vi "Initialize.vi"(7 "Serial Configuration":T1={"Baud Rate"=9600, "Parity"=0, "Data Bits"=8, "Stop Bits"=10, "Flow Control"=0} {"Flow Control" items=["None", "XON/XOFF", "RTS/CTS", "XON/XOFF & RTS/CTS", "DTR/DSR", "XON/XOFF & DTR/DSR"]; "Stop Bits" items=["1.0"=10, "1.5"=15, "2.0"=20]; "Data Bits" items=["7"=7, "8"=8]; "Parity" items=["None", "Odd", "Even", "Mark", "Space"]; "Baud Rate" items=["300"=300, "600"=600, "1200"=1200, "2400"=2400, "4800"=4800, "9600"=9600, "19200"=19200]}, 8 "error in (no error)":errorcluster, 9 "Reset (True)":bool=TRUE, 10 "ID Query (True)":bool=TRUE, 11 "VISA resource name":refnum<visa-resource-name>) -> (0 "error out":errorcluster, 3 "VISA resource name out":refnum<visa-resource-name>)   [LabVIEW 2020, in "Keithley 24XX.lvlib"]
doc: "Establishes communication with the instrument and optionally performs an instrument identification query and/or an instrument reset. It also places the instrument in a default state needed for other instrument driver operations. Therefore, call this VI before calling other instrument driver VIs for this instrument. Generally, you need to call the Initialize VI only once at the beginning of an application."
uses:
  Keithley 24XX.lvlib
panel:
  # "(c) 2006 - 2015 National Instruments.  ALL RIGHTS RESERVED."
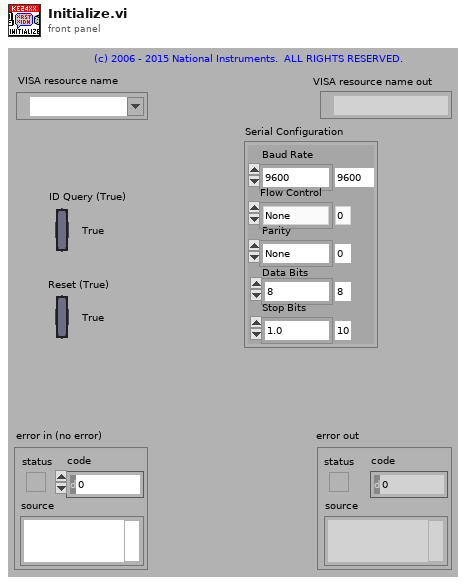
[diagram p1: front panel]
types:
  T1 = cluster{"Baud Rate":u32, "Parity":u16, "Data Bits":u16, "Stop Bits":u16, "Flow Control":u16}
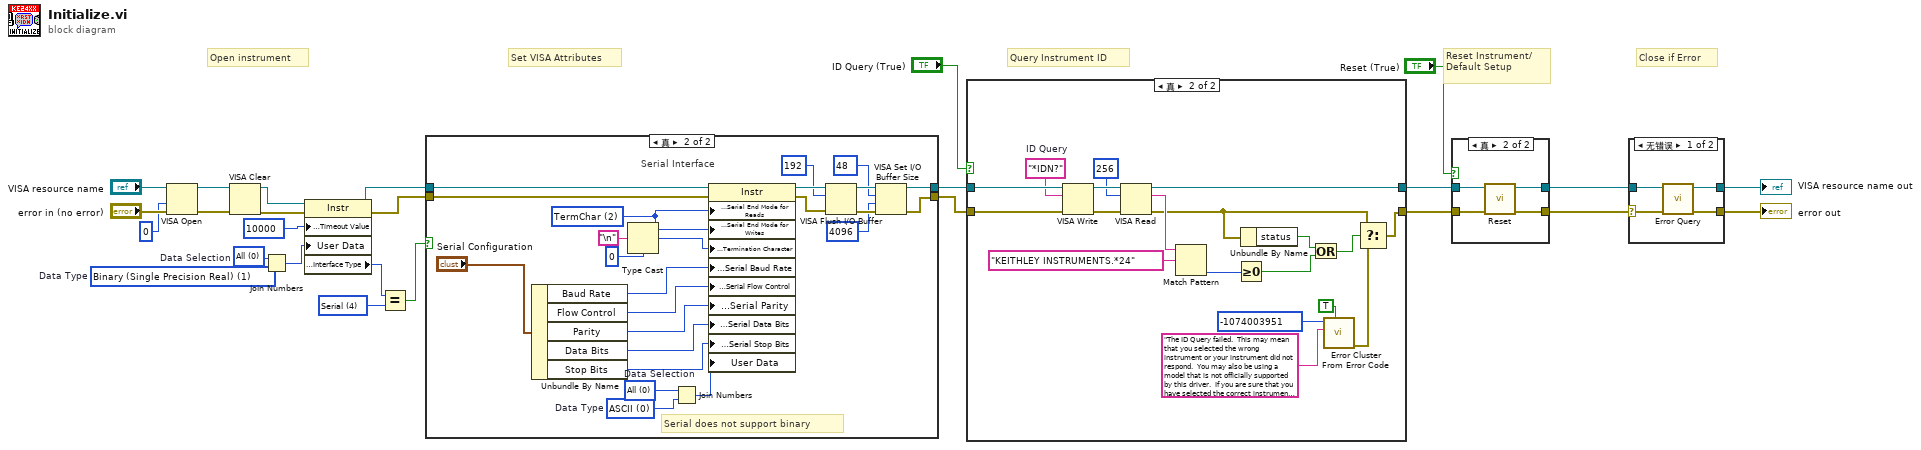
[diagram p0: block diagram]
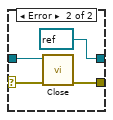
[diagram p3: hidden frame]
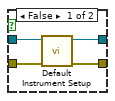
[diagram p4: hidden frame]
diagram:
  w2 = u16 1 items=["ASCII", "Binary (Single Precision Real)"]  # Data Type
  w3 = u16 0 items=["All", "Volt and Amp", "Volt", "Amp"]  # Data Selection
  w14 = u16 4 items=["GPIB"=1, "VXI"=2, "GPIB-VXI"=3, "Serial"=4, "PXI"=5, "TCPIP"=6, "USB"=7] ("Interface Information:Interface Type")
  # "Set VISA Attributes"
  # "Close if Error"
  # "Query Instrument ID"
  # "Reset Instrument/\nDefault Setup"
  # "Open instrument"
  n1 = VISA Open(access mode=u32 0, error in (no error)="error in (no error)", VISA resource name="VISA resource name") -> (VISA resource name=w12:refnum<visa-resource-name>, error out=w11:errorcluster)  [unwired: 2 in]
  n2 = VISA Clear(VISA resource name=w12, error in (no error)=w11) -> (VISA resource name out=w10:refnum<visa-resource-name>, error out=w9:errorcluster)
  n3 = Join Numbers(hi=w3, lo=w2) -> ((hi.lo)=w1:u32)
  n4 = property class="Instr"(reference=w10, error in=w9, "General Settings:Timeout Value"=u32 10000, "User Data"=w1) -> (reference out=w17:refnum<visa-resource-name>, error out=w16:errorcluster, "Interface Information:Interface Type"=w4:u16)
  n5 = Equal?(x=w4, y=w14) -> (x = y?=w15:bool)
  n6 = case shown="真" w15 {
    tunnel: [w27 w49] -> w19
    tunnel: [w28 w46] -> w18
    tunnel: w17 -> [w27 w51]
    tunnel: w16 -> [w28 w52]
    frame False {
      # "GPIB"
    }
    frame True {
      w31 = u16 0 items=["ASCII", "Binary (Single Precision Real)"]  # Data Type
      w29 = u16 0 items=["All", "Volt and Amp", "Volt", "Amp"]  # Data Selection
      w39 = u16 2 items=["None", "LastBit", "TermChar"] ("Serial Settings:Serial End Mode for Reads")
      # "Serial does not support binary"
      # "Serial Interface"
      n7 = Unbundle By Name("Serial Configuration") -> ("Baud Rate"=w37:u32, "Flow Control"=w33:u16, "Parity"=w35:u16, "Data Bits"=w36:u16, "Stop Bits"=w32:u16)
      n8 = Type Cast(type=u8 0, x="\n" ("Line Feed Constant")) -> (*(type *) &x=w38:u8)
      n9 = Join Numbers(hi=w29, lo=w31) -> ((hi.lo)=w30:u32)
      n10 = property class="Instr"(reference=w51, error in=w52, "Serial Settings:Serial End Mode for Reads"=w39, "Serial Settings:Serial End Mode for Writes"=w39, "Message Based Settings:Termination Character"=w38, "Serial Settings:Serial Baud Rate"=w37, "Serial Settings:Serial Flow Control"=w33, "Serial Settings:Serial Parity"=w35, "Serial Settings:Serial Data Bits"=w36, "Serial Settings:Serial Stop Bits"=w32, "User Data"=w30) -> (reference out=w45:refnum<visa-resource-name>, error out=w48:errorcluster)
      n11 = VISA Flush I/O Buffer(VISA resource name=w45, mask (16)=u16 192, error in (no error)=w48) -> (VISA resource name out=w50:refnum<visa-resource-name>, error out=w47:errorcluster)
      n12 = VISA Set I/O Buffer Size(VISA resource name=w50, mask (16)=u16 48, size (4096)=u32 4096 ("size (0)"), error in (no error)=w47) -> (VISA resource name out=w49:refnum<visa-resource-name>, error out=w46:errorcluster)
    }
  }
  n13 = case shown="真" "ID Query (True)" {
    tunnel: [w53 w73] -> w25
    tunnel: [w54 w70] -> w26
    tunnel: w19 -> [w54 w71]
    tunnel: w18 -> [w53 w72]
    frame False {
    }
    frame True {
      w64 = "*IDN?"  # ID Query
      n14 = VISA Write(VISA resource name=w71, write buffer=w64, error in (no error)=w72) -> (VISA resource name out=w68:refnum<visa-resource-name>, error out=w67:errorcluster)  [unwired: 1 out]
      n15 = VISA Read(VISA resource name=w68, byte count=u32 256, error in (no error)=w67) -> (VISA resource name out=w70:refnum<visa-resource-name>, read buffer=w69:string, error out=w58:errorcluster)  [unwired: 1 out]
      n16 = Match Pattern(string=w69, regular expression="KEITHLEY INSTRUMENTS.*24") -> (offset past match=w59:i32)  [unwired: 1 in, 3 out]
      n17 = Greater Or Equal To 0?(x=w59) -> (x >= 0?=w56:bool)
      n18 = Unbundle By Name(w58) -> ("status"=w57:bool)
      n19 = Or(x=w57, y=w56) -> (x .or. y?=w55:bool)
      n20 = call <vilib>:"Error Cluster From Error Code.vi"("show call chain? (False)"=TRUE, "error message (\"\")"="The ID Query failed.  This may mean that you selected the wrong instrument or your instrument did not respond.  You may also be using a model that is not officially supported by this driver.  If you are sure that you have selected the correct instrument and it is responding, try disabling the ID Query." ("Source (VI Name)"), "error code (0)"=-1074003951 ("Code")) -> ("error out"=w63:errorcluster)  [unwired: 6 in]
      n21 = Select(t=w58, s=w55, f=w63) -> (s? t:f=w73:errorcluster)
    }
  }
  n22 = case shown="真" "Reset (True)" {
    tunnel: w25 -> [w76 w78]
    tunnel: [w75 w81] -> w5
    tunnel: w26 -> [w77 w79]
    tunnel: [w74 w80] -> w6
    frame False {
      n23 = call "Default Instrument Setup.vi"("error in (no error)"=w76, "VISA resource name"=w77) -> ("error out"=w75:errorcluster, "VISA resource name out"=w74:refnum<visa-resource-name>)  [unwired: 8 in]
    }
    frame True {
      n24 = call "Reset.vi"("error in (no error)"=w78, "VISA resource name"=w79) -> ("error out"=w81:errorcluster, "VISA resource name out"=w80:refnum<visa-resource-name>)  [unwired: 8 in]
    }
  }
  n25 = case shown="无错误" w5 {
    selector: w5 -> [w83 w87]
    tunnel: w6 -> [w82 w88]
    tunnel: [w85 refnum<visa-resource-name> refnum ("VISA resource name out")] -> w8
    tunnel: [w84 w89] -> w7
    frame No Error {
      n26 = call "Error Query.vi"("error in (no error)"=w83, "VISA resource name"=w82) -> ("error out"=w84:errorcluster, "VISA resource name out"=w85:refnum<visa-resource-name>)  [unwired: 6 in, 2 out]
    }
    frame Error {
      n27 = call "Close.vi"("error in (no error)"=w87, "VISA resource name"=w88) -> ("error out"=w89:errorcluster)  [unwired: 9 in]
    }
  }
  "VISA resource name out" <- w8
  "error out" <- w7
